vi "http handle content data.vi"(4 "transmit queue":refnum<queue>, 6 "exec queue":refnum<queue>, 9 "server properties":T1={"max url size"=8000, "max header"=8000, "timeout ms"=5000, "max data size"=104857600}, 10 "application request":T2, 11 "TCP Network Connection in":refnum<k5>) -> (3 "abort":bool)   [LabVIEW 2013]
uses:
  http request.ctl
  http method.ctl
  http response.ctl
  http response packet type.ctl
  http server properties.ctl
  http chunked encoding state.ctl
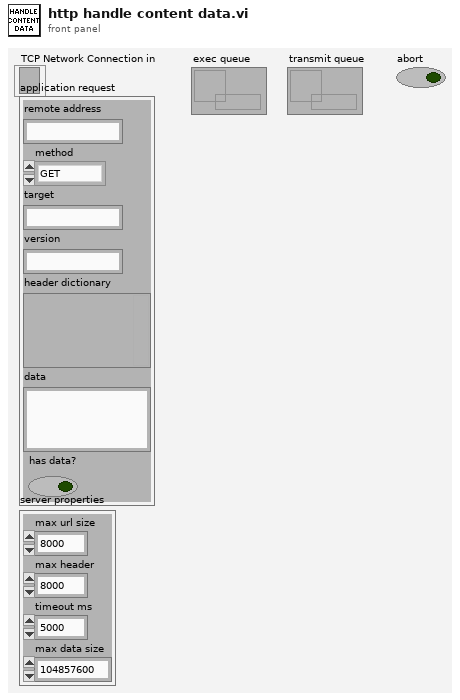
[diagram p1: front panel]
types:
  T1 = typedef "http server properties.ctl" = cluster{"max url size":i32, "max header":i32, "timeout ms":i32, "max data size":i32}
  T2 = typedef "http request.ctl" = cluster{"remote address":string, "method":T3, "target":string, "version":string, "header dictionary":variant, "data":string, "has data?":bool}
  T3 = typedef "http method.ctl" = enum16{"GET", "POST", "PUT", "DELETE", "HEAD", "OPTIONS", "upgrade"}
  T4 = typedef "http chunked encoding state.ctl" = enum16{"length", "data", "trailer"}
  T5 = enum16{"Standard", "Buffered", "CRLF", "Immediate"}
  T6 = typedef "http response.ctl" = cluster{"packet type":T7, "reason code":u16, "status string":string, "header dictionary":variant, "cookies":string[], "data":string}
  T7 = typedef "http response packet type.ctl" = enum16{"full response", "header only", "data only", "last data"}
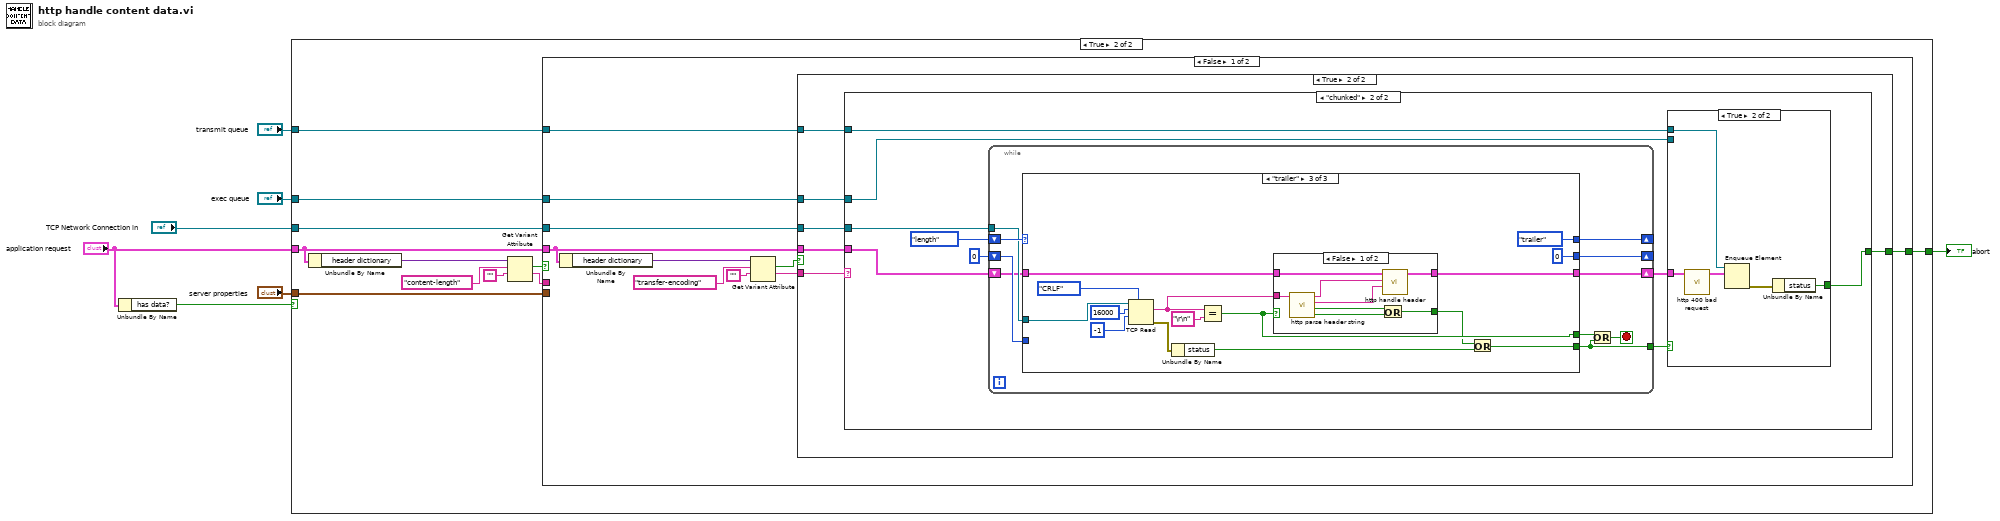
[diagram p0: block diagram]
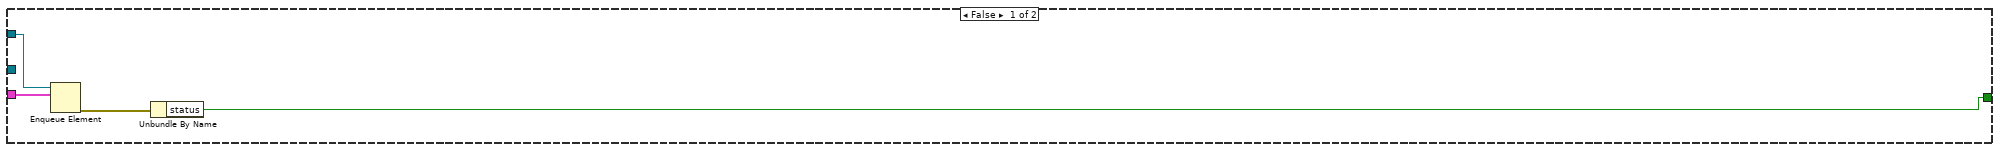
[diagram p2: hidden frame]
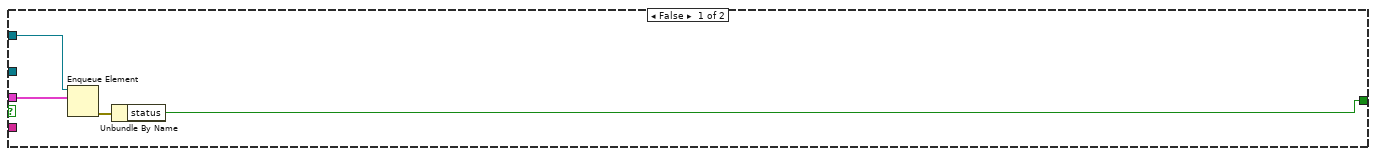
[diagram p3: hidden frame]
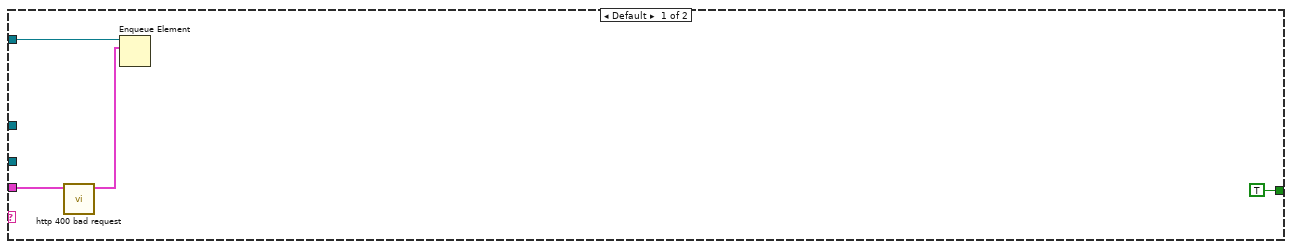
[diagram p4: hidden frame]
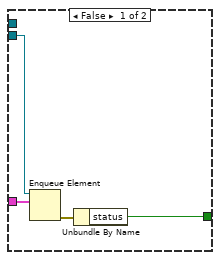
[diagram p5: hidden frame]
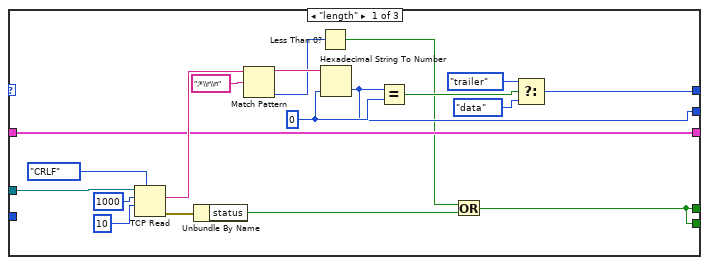
[diagram p6: hidden frame]
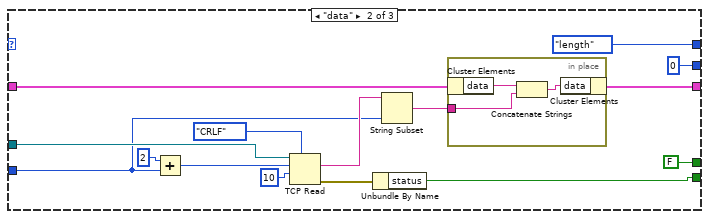
[diagram p7: hidden frame]
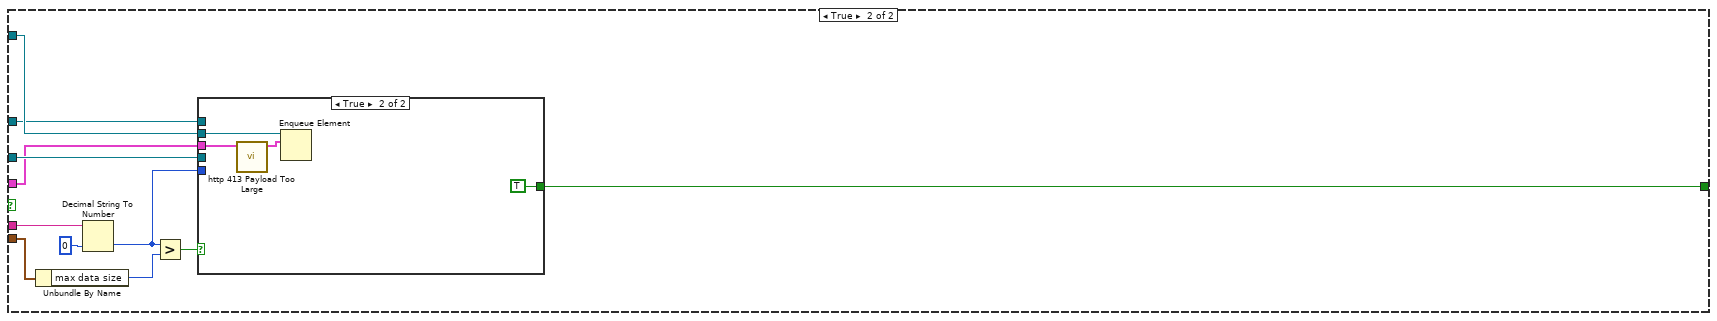
[diagram p9: hidden frame]
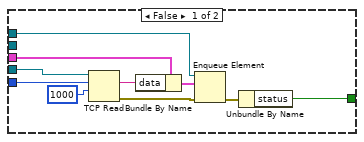
[diagram p10: hidden frame]
diagram:
  n1 = Unbundle By Name("application request") -> ("has data?"=w1:bool)
  n2 = case shown="True" w1 {
    tunnel: "TCP Network Connection in" -> [_ w22]
    tunnel: [w8 w21] -> w6
    tunnel: "server properties" -> [_ w20]
    tunnel: "transmit queue" -> [_ w19]
    tunnel: "exec queue" -> [w10 w18]
    tunnel: "application request" -> [w11 w12]
    frame False {
      n3 = Enqueue Element(queue=w10, element=w11) -> (error out=w9:errorcluster)  [unwired: 2 in, 2 out]
      n4 = Unbundle By Name(w9) -> ("status"=w8:bool)
    }
    frame True {
      n5 = Unbundle By Name(w12) -> ("header dictionary"=w13:variant)
      n6 = Get Variant Attribute(Variant=w13, name="content-length", default value (empty Variant)="") -> (found=w16:bool, value=w17:string)  [unwired: 1 in, 2 out]
      n7 = case shown="False" w16 {
        tunnel: w17 -> [_ w146]
        tunnel: w12 -> [w26 w142]
        tunnel: w22 -> [w25 w144]
        tunnel: [w28 w143] -> w21
        tunnel: w20 -> [_ w141]
        tunnel: w19 -> [w23 w137]
        tunnel: w18 -> [w24 w136]
        frame False {
          n8 = Unbundle By Name(w26) -> ("header dictionary"=w32:variant)
          n9 = Get Variant Attribute(Variant=w32, name="transfer-encoding", default value (empty Variant)="") -> (found=w27:bool, value=w29:string)  [unwired: 1 in, 2 out]
          n10 = case shown="True" w27 {
            tunnel: w29 -> [_ w42]
            tunnel: [w33 w41] -> w28
            tunnel: w26 -> [w36 w40]
            tunnel: w25 -> [_ w39]
            tunnel: w24 -> [w35 w38]
            tunnel: w23 -> [_ w37]
            frame False {
              n11 = Enqueue Element(queue=w35, element=w36) -> (error out=w34:errorcluster)  [unwired: 2 in, 2 out]
              n12 = Unbundle By Name(w34) -> ("status"=w33:bool)
            }
            frame True {
              n13 = case shown="\"chunked\"" w42 {
                tunnel: [TRUE w48] -> w41
                tunnel: w40 -> [w43 w52]
                tunnel: w39 -> [_ w54]
                tunnel: w38 -> [_ w49]
                tunnel: w37 -> [w44 w47]
                frame Default {
                  n14 = call "http 400 bad request.vi"("application request in"=w43) -> ("application request out"=w45:T6)  [unwired: 10 in]
                  n15 = Enqueue Element(queue=w44, element=w45) -> ()  [unwired: 2 in, 3 out]
                }
                frame "chunked" {
                  n16 = while {
                    shift-right: [w72] -> _
                    shift-left: http_chunked_encoding_state."length" -> [w74]
                    tunnel: w54 -> [w73]
                    shift-right: [w70] -> _
                    shift-left: 0 ("default (0 I32)") -> [w69]
                    shift-right: [w67] -> w50
                    shift-left: w52 -> [w68]
                    tunnel: [w65] -> w51
                    stop <- w66 stop-if-true
                    n17 = case shown="\"trailer\"" w74 {
                      tunnel: w73 -> [w93 w106 w123]
                      tunnel: [w80 http_chunked_encoding_state."length" http_chunked_encoding_state."trailer"] -> w72
                      tunnel: [w76 FALSE w117] -> w71
                      tunnel: [w85 0 0] -> w70
                      tunnel: w69 -> [_ w102 _]
                      tunnel: w68 -> [w79 w95 w115]
                      tunnel: [w79 w94 w116] -> w67
                      tunnel: [w76 w96 w114] -> w65
                      frame "length" {
                        w86 = 0 ("default (0 I32)")
                        n18 = TCP Read(connection ID=w93, bytes to read=1000, 7:T5."CRLF" ("mode (standard)"), 9:10 ("timeout ms (25000)")) -> (data out=w89:string, error out=w77:errorcluster)  [unwired: 1 in, 1 out]
                        n19 = Unbundle By Name(w77) -> ("status"=w75:bool)
                        n20 = Match Pattern(string=w89, regular expression=";*\\r\\n") -> (before substring=w87:string, offset past match=w84:i32)  [unwired: 1 in, 2 out]
                        n21 = Less Than 0?(x=w84) -> (x < 0?=w78:bool)
                        n22 = Hexadecimal String To Number(string=w87, default (0uL)=w86) -> (number=w85:i32)  [unwired: 1 in, 1 out]
                        n23 = Equal?(x=w85, y=w86) -> (x = y?=w83:bool)
                        n24 = Or(x=w78, y=w75) -> (x .or. y?=w76:bool)
                        n25 = Select(t=http_chunked_encoding_state."trailer", s=w83, f=http_chunked_encoding_state."data") -> (s? t:f=w80:T4)
                      }
                      frame "data" {
                        n26 = Add(x=2, y=w102) -> (x+y=w105:i32)
                        n27 = TCP Read(connection ID=w106, bytes to read=w105, 7:T5."CRLF" ("mode (standard)"), 9:10 ("timeout ms (25000)")) -> (data out=w103:string, error out=w97:errorcluster)  [unwired: 1 in, 1 out]
                        n28 = Unbundle By Name(w97) -> ("status"=w96:bool)
                        n29 = String Subset(string=w103, length (rest)=w102) -> (substring=w101:string)  [unwired: 1 in]
                        n30 = in-place {
                          in-place-border: w101 -> [w111]
                          n31 = in-place-cluster #1(w95) -> ("data"=w110:string)
                          n32 = Concatenate Strings(w110, w111) -> (w109:string)
                          n33 = in-place-cluster #1("data"=w109) -> (w94:T2)
                        }
                      }
                      frame "trailer" {
                        n34 = TCP Read(connection ID=w123, bytes to read=16000, 7:T5."CRLF" ("mode (standard)"), 9:-1 ("timeout ms (25000)")) -> (data out=w112:string, error out=w121:errorcluster)  [unwired: 1 in, 1 out]
                        n35 = Unbundle By Name(w121) -> ("status"=w120:bool)
                        n36 = Equal?(x=w112, y="\r\n" ("x")) -> (x = y?=w117:bool)
                        n37 = case shown="False" w117 {
                          tunnel: [w134 w135] -> w116
                          tunnel: w115 -> [w133 w135]
                          tunnel: [w129 _] -> w113
                          tunnel: w112 -> [w130 _]
                          frame False {
                            n38 = call "http parse header string.vi"("raw string"=w130) -> ("no field name"=w128:bool, "no crlf"=w132:bool, "header field data"=w131:string, "header field name"=w127:string)  [unwired: 7 in]
                            n39 = Or(x=w132, y=w128) -> (x .or. y?=w129:bool)
                            n40 = call "http handle header.vi"("header field data"=w131, "header field name"=w127, "application request in"=w133) -> ("application request out"=w134:T2)  [unwired: 8 in]
                          }
                          frame True {
                          }
                        }
                        n41 = Or(x=w113, y=w120) -> (x .or. y?=w114:bool)
                      }
                    }
                    n42 = Or(x=w71, y=w65) -> (x .or. y?=w66:bool)
                  }
                  n43 = case shown="True" w51 {
                    tunnel: w50 -> [w58 w62]
                    tunnel: w49 -> [w59 _]
                    tunnel: [w56 w63] -> w48
                    tunnel: w47 -> [_ w60]
                    frame False {
                      n44 = Enqueue Element(queue=w59, element=w58) -> (error out=w57:errorcluster)  [unwired: 2 in, 2 out]
                      n45 = Unbundle By Name(w57) -> ("status"=w56:bool)
                    }
                    frame True {
                      n46 = call "http 400 bad request.vi"("application request in"=w62) -> ("application request out"=w61:T6)  [unwired: 10 in]
                      n47 = Enqueue Element(queue=w60, element=w61) -> (error out=w64:errorcluster)  [unwired: 2 in, 2 out]
                      n48 = Unbundle By Name(w64) -> ("status"=w63:bool)
                    }
                  }
                }
              }
            }
          }
        }
        frame True {
          n49 = Unbundle By Name(w141) -> ("max data size"=w140:i32)
          n50 = Decimal String To Number(string=w146, default (0L)=0 ("default (0 I32)")) -> (number=w139:i32)  [unwired: 1 in, 1 out]
          n51 = Greater?(x=w139, y=w140) -> (0:w138:bool)
          n52 = case shown="True" w138 {
            tunnel: w144 -> [w156 _]
            tunnel: [w154 TRUE ("status")] -> w143
            tunnel: w142 -> [w153 w159]
            tunnel: w139 -> [w150 _]
            tunnel: w137 -> [_ w157]
            tunnel: w136 -> [w148 _]
            frame False {
              n53 = TCP Read(connection ID=w156, bytes to read=w150, 9:1000 ("timeout ms (25000)")) -> (data out=w152:string, error out=w151:errorcluster)  [unwired: 2 in, 1 out]
              n54 = Bundle By Name(cluster=w153, "data"=w152) -> (w147:T2)
              n55 = Enqueue Element(queue=w148, element=w147, error in (no error)=w151) -> (error out=w149:errorcluster)  [unwired: 1 in, 2 out]
              n56 = Unbundle By Name(w149) -> ("status"=w154:bool)
            }
            frame True {
              n57 = call "http 413 Payload Too Large.vi"("application request in"=w159) -> ("application request out"=w158:T6)  [unwired: 10 in]
              n58 = Enqueue Element(queue=w157, element=w158) -> ()  [unwired: 2 in, 3 out]
            }
          }
        }
      }
    }
  }
  "abort" <- w6
